vi "GV_uTTA_Configuration.vi"() -> ()   [LabVIEW 2021]
panel:
  in  "Channel_Name_Max_Length":u32=30
  in  "DUT_Name_Max_Length":u32=50
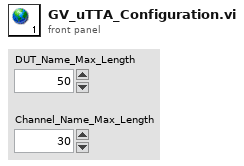
[diagram p1: front panel]
diagram:
